vi "FdxCmdMonQueueControlCvi.vi"(6 "MaxFileSize":u32, 7 "RecordingFileName":path, 8 "error in":errorcluster, 9 "QueueCtrl":u32(ring) items=["FDX_MON_QUEUE_CREATE", "FDX_MON_QUEUE_DELETE"], 10 "QueueId":u32, 11 "InstrumentHandle_port":u32) -> (0 "error out":errorcluster, 1 "GlobMonSize":u32, 2 "QueueIdOut":u32, 3 "InstrumentHandle_port":u32)   [LabVIEW 2020, in "AIM664LV.lvlib"]
doc: "This function controls creation or deletion of queues, associated with the chronological monitor. The function returns a queue ID which must be used for all queue related functions.\nOperating mode must be defined by using AiFdxCmdRxModeControl and AiFdxCmdCaptureControl before using this function. Dependant on the capture mode, the Frame data will be buffered in a second level queue of the onboard Target-Software (FDX_MON_CONTINUOUS and FDX_MON_RECORDING). In other cases the frames will be read directly from the receive buffer."
uses:
  AIM664LV.lvlib
  AFDX_LibraryAdmin/FdxGlobalDllPath.vi
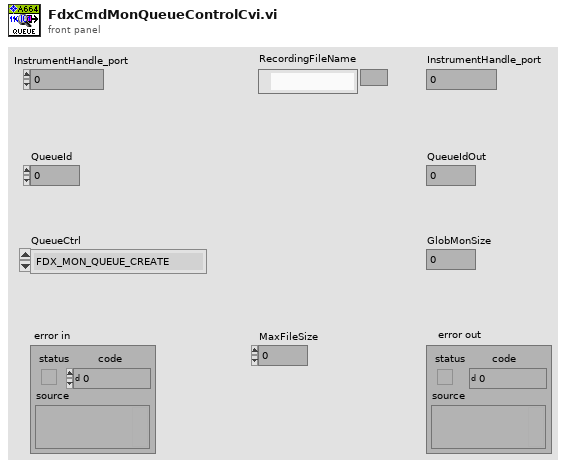
[diagram p1: front panel]
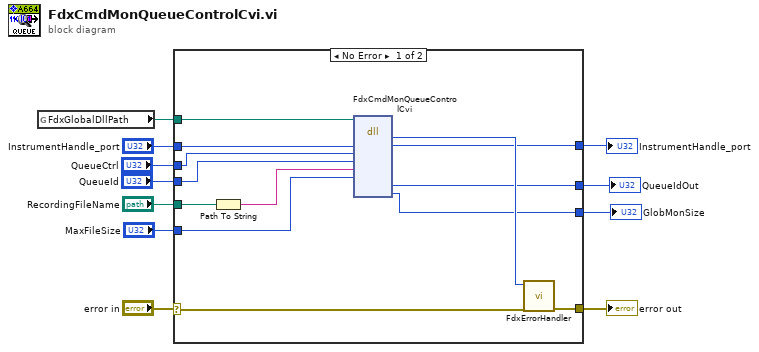
[diagram p0: block diagram]
diagram:
  n1 = global read "FdxGlobalDllPath.vi" "FdxGlobalDllPath"() -> (w9:path)
  n2 = case shown="No Error" "error in" {
    selector: "error in" -> [w23 w26]
    tunnel: [w24 w26] -> w11
    tunnel: w9 -> [w21 _]
    tunnel: "InstrumentHandle_port" -> [w20 w25]
    tunnel: [w19 w25] -> w7
    tunnel: [w18 _] -> w6
    tunnel: [w17 _] -> w5
    tunnel: "QueueId" -> [w15 _]
    tunnel: "RecordingFileName" -> [w13 _]
    tunnel: "QueueCtrl" -> [w16 _]
    tunnel: "MaxFileSize" -> [w14 _]
    frame No Error {
      n3 = Path To String(path=w13) -> (string=w12:string)
      n4 = dll-call lib="aim_fdx.19.dll" fn="FdxCmdMonQueueControlCvi"(path in=w21, "InstrumentHandle"=w20, "QueueCtrl"=w16, "QueueId"=w15, "RecordingFileName"=w12, "MaxFileSize"=w14) -> ("status"=w22:i32, "InstrumentHandle"=w19:u32, "QueueIdOut"=w18:u32, "GlobMonSize"=w17:u32)  [unwired: 7 in, 3 out]
      n5 = call "FdxErrorHandler.vi"("error in"=w23, "AIM Error"=w22) -> ("error out"=w24:errorcluster)  [unwired: 9 in]
    }
    frame Error {
    }
  }
  "error out" <- w11
  "InstrumentHandle_port" <- w7
  "QueueIdOut" <- w6
  "GlobMonSize" <- w5
